vi "Avantes - AVS_GetSaturatedPixels.vi"(8 "error in (no error)":errorcluster, 11 "AVS Settings In":T1) -> (0 "error out":errorcluster, 1 "a_pSaturated":u8[](array[numeric]), 2 "Saturated?":bool, 3 "AVS Settings Out":T1)   [LabVIEW 2013, in "AvaSpec.lvlib" / "Avantes Spectrometer Functions.lvlib"]
uses:
  Avantes Spectrometer Functions.lvlib
  AVS settings.ctl
  AvaSpec.lvlib
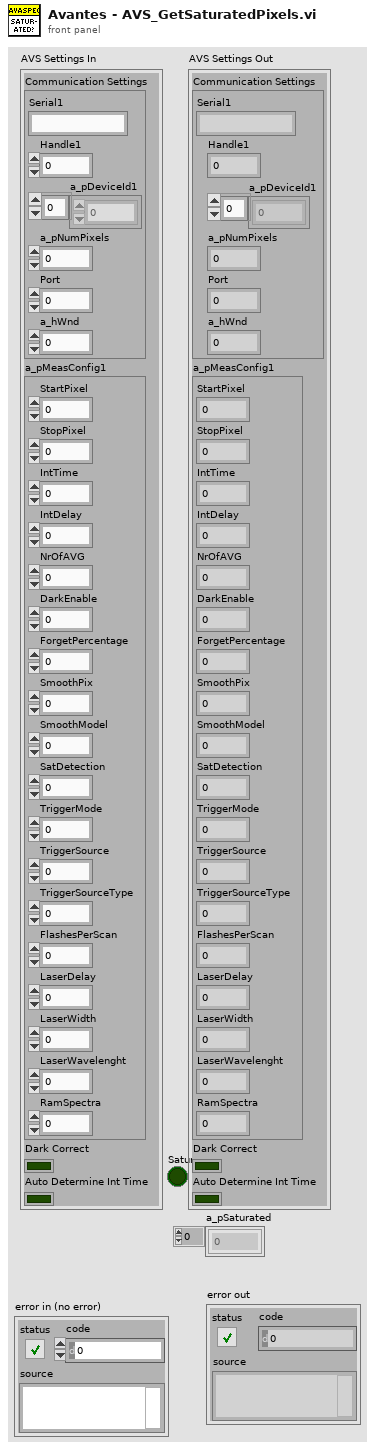
[diagram p1: front panel]
types:
  T1 = typedef "AvaSpec.lvlib/AVS settings.ctl" = cluster{"Communication Settings":cluster{"Serial1":string, "Handle1":i32, "a_pDeviceId1":u8[], "a_pNumPixels":u16, "Port":i32, "a_hWnd":i32}, "a_pMeasConfig1":cluster{"StartPixel":u16, "StopPixel":u16, "IntTime":sgl, "IntDelay":u32, "NrOfAVG":u32, "DarkEnable":u8, "ForgetPercentage":u8, "SmoothPix":u16, "SmoothModel":u8, "SatDetection":u8, "TriggerMode":u8, "TriggerSource":u8, "TriggerSourceType":u8, "FlashesPerScan":u16, "LaserDelay":u32, "LaserWidth":u32, "LaserWavelenght":sgl, "RamSpectra":u16}, "Dark Correct":bool, "Auto Determine Int Time":bool}
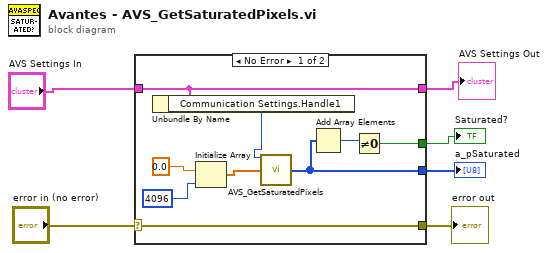
[diagram p0: block diagram]
diagram:
  n1 = case shown="No Error" "error in (no error)" {
    selector: "error in (no error)" -> [w7 w17]
    tunnel: [w15 w16] -> w1
    tunnel: "AVS Settings In" -> [w15 w16]
    tunnel: [w7 w17] -> w5
    tunnel: [w10 _] -> w4
    tunnel: [w8 _] -> w3
    frame No Error {
      n2 = Unbundle By Name(w15) -> ("Communication Settings.Handle1"=w14:i32)
      n3 = Initialize Array(0.0 ("element"), 4096 ("dimension size")) -> (w11:dbl[])
      n4 = call "AVS_GetSaturatedPixels.vi"("a_hDevice"=w14, "a_pSaturated"=w11) -> ("a_pSaturated"=w10:u8[])  [unwired: 12 in, 1 out]
      n5 = Add Array Elements(numeric array=w10) -> (sum=w9:u8)
      n6 = Not Equal To 0?(x=w9) -> (x != 0?=w8:bool)
    }
    frame Error {
    }
  }
  "error out" <- w5
  "a_pSaturated" <- w4
  "Saturated?" <- w3
  "AVS Settings Out" <- w1
